vi "2 OnePointOfSailGoodness.vi"(4 "Heading to Test":dbl) -> (1 "Goodness":dbl)   [LabVIEW 2011]
doc: "Takes the absolute wind vector, the heading of your next waypoint, and a test heading and outputs a goodness value for the test heading. The criteria is the speed to get to the waypoint.\n\nThe goodness is evaluated by taking the softmax of an angle with all possible complimenting angles (i.e. if the test heading is 10 degrees it is matched with -1 through -89; note that angles are adjusted to be degrees from directly at the waypoint). The specific calculation for finding the net velocity of a pair of angles requires the velocities from the polar plot."
uses:
  2 Typedefs/absolute wind direction.ctl
  2 Globals/2 TuningConstants.vi
  2 Globals/2 Global.vi
panel:
  out "Desired Apparent Wind\nDirection (º)":T1
  # "Inputs"
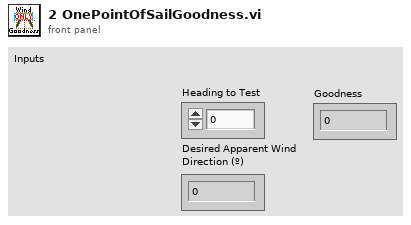
[diagram p1: front panel]
types:
  T1 = typedef "absolute wind direction.ctl" = dbl
  T2 = typedef "Apparent Wind Mode.ctl" = cluster{"Desired Apparent\nWind Direction":dbl, "On":bool}
  T3 = typedef "apparent wind direction.ctl" = dbl
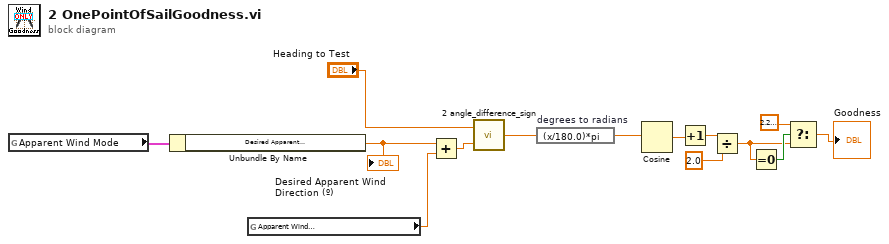
[diagram p0: block diagram]
diagram:
  n1 = global read "2 TuningConstants.vi" "Apparent Wind Mode"() -> (w5:T2)
  n2 = Unbundle By Name(w5) -> ("Desired Apparent\nWind Direction"=w2:dbl)
  "Desired Apparent Wind\nDirection (º)" <- w2
  n3 = global read "2 Global.vi" "Apparent Wind\nDirection (º)"() -> (w1:T3)
  n4 = Add(x=w2, y=w1) -> (x+y=w3:T3)
  n5 = call "2 angle_difference_sign.vi"("Angle 2"=w3, "Angle 1"="Heading to Test") -> ("Difference"=w11:dbl)
  n6 = expression code="(x/180.0)*pi" "degrees to radians"(w11) -> (w12:dbl)
  n7 = Cosine(x=w12) -> (cos(x)=w10:dbl)
  n8 = Increment(x=w10) -> (x+1=w9:dbl)
  n9 = Divide(x=w9, y=2.0) -> (x/y=w7:dbl)
  n10 = Equal To 0?(x=w7) -> (x = 0?=w13:bool)
  n11 = Select(t=2.220446049250313e-16, s=w13, f=w7) -> (s? t:f=→"Goodness":dbl)
